vi "ME135_Project_Final.vi"() -> ()   [LabVIEW 2021]
doc: "This example performs writes and reads on a serial port, as directed by the user. You can press the Write and Read buttons, and change the Read Count, while the example is running.\n\nThe parameters set for the serial port must match the parameters of the connected instrument or device. In this example, the Read Count parameter specifies the number of bytes that the serial port reads. If there were more bytes at the port than the specified number, those bytes would not be read. If there were less bytes at the port than the specified number, you would receive a timeout error.\n\nThis example expands upon the flow control options for XON and XOFF, allowing the user to choose those control characters. Also, the user can enable or disable a termination character. Some devices require a termination character in order to identify the end of command strings. Some devices send a termination character to signify the end of data to be read. This example shows how you can end the Read operation once a termination character is detected in the buffer and/or append a termination character at the end of the Write data."
uses:
  Serial - Settings.ctl
  Serial - XON-XOFF Characters.ctl
  Serial - ASCII Characters-1.ctl
  ESP32-PSOC-State Machine.ctl
  <vilib>/Instr/_visa.llb/VISA Flush IO Buffer Mask.ctl
  <vilib>/Instr/_visa.llb/VISA Configure Serial Port (Instr).vi
panel:
  in  "Toggle Motors":bool
  out "Backward":bool
  out "Right":bool
  out "Left":bool
  out "Forward":bool
  out "Obstacle Detected":bool
  out "error":bool=TRUE
  out "Connected":bool
  out "Serial Settings:Number of Bytes at Serial Port":u32
  out "Response 2":string="Exiting LabVIEW"
  in  "Turn On":bool
  in  "Enum":T1
  in  "Termination Character":u8=10 format="%.0x"
  in  "End Write on Termination Character?":bool=TRUE
  in  "Exit Labview":bool
  out "Read Count":u32=1000
  out "Response":string
  in  "XON/XOFF Characters":T2={"XON"=enum."DC1", "XOFF"=enum."DC3"}
  in  "Serial Settings":T4={"baud rate"=115200, "data bits"=8, "parity"=enum."None", "stop bits"=10, "flow control"=0} {"flow control" items=["None"=0, "XON/XOFF"=1, "RTS/CTS"=2, "DTR/DSR"=4]; "stop bits" items=["1.0"=10, "1.5"=15, "2.0"=20]; "data bits" min=5 max=8 step=1; "baud rate" items=["75"=75, "110"=110, "134"=134, "150"=150, "300"=300, "600"=600, "1200"=1200, "1800"=1800, "2400"=2400, "4800"=4800, "7200"=7200, "9600"=9600, "14400"=14400, "19200"=19200, "28800"=28800, "38400"=38400, "56000"=56000, "57600"=57600, "115200"=115200, "128000"=128000, "230400"=230400]}
  in  "End Read on Termination Character?":bool=TRUE
  in  "VISA resource name":refnum<visa-resource-name>="COM8"
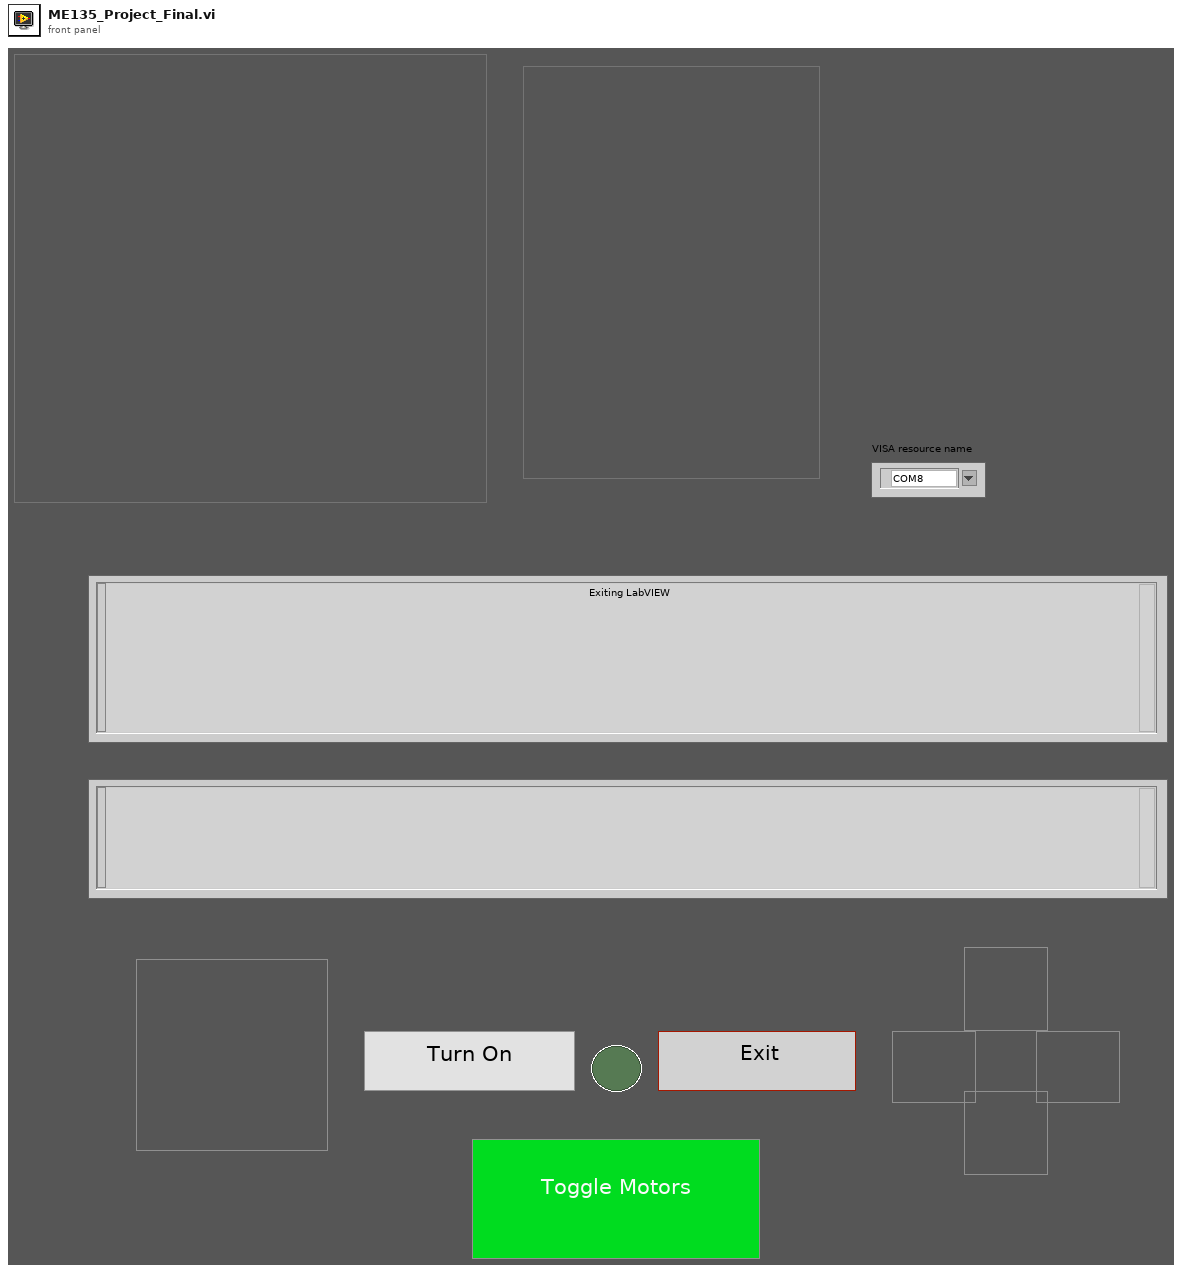
[diagram p1: front panel]
types:
  T1 = typedef "ESP32-PSOC-State Machine.ctl" = enum8{"Init", "Connect", "idle", "send", "wait", "receive", "que", "error", "exit"}
  T2 = typedef "Serial - XON-XOFF Characters.ctl" = cluster{"XON":T3, "XOFF":T3}
  T3 = typedef "Serial - ASCII Characters-1.ctl" = enum16{"NUL", "SOH", "STX", "ETX", "EOT", "ENQ", "ACK", "BEL", "BS", "HT", "LF", "VT", "FF", "CR", "SO", "SI", "DLE", "DC1", "DC2", "DC3", "DC4", "NAK", "SYN", "ETB", "CAN", "EM", "SUB", "ESC", "FS", "GS", "RS", "US", "SP", "!", "\"", "#", "$", "%", "&", "'", "(", ")", "*", "+", ",", "- (-)", ".", "/", "0", "1", "2", "3", "4", "5", "6", "7", "8", "9", ":", ";", "<", "=", ">", "?", "@", "A", "B", "C", "D", "E", "F", "G", "H", "I", "J", "K", "L", "M", "N", "O", "P", "Q", "R", "S", "T", "U", "V", "W", "X", "Y", "Z", "[", "\\", "]", "^", "_", "`", "a", "b", "c", "d", "e", "f", "g", "h", "i", "j", "k", "l", "m", "n", "o", "p", "q", "r", "s", "t", "u", "v", "w", "x", "y", "z", "{", "|", "}", "~"}
  T4 = typedef "Serial - Settings.ctl" = cluster{"baud rate":u32, "data bits":u16, "parity":enum16{"None", "Odd", "Even", "Mark", "Space"}, "stop bits":u16, "flow control":u16}
  T5 = typedef "VISA Flush IO Buffer Mask.ctl" = u16
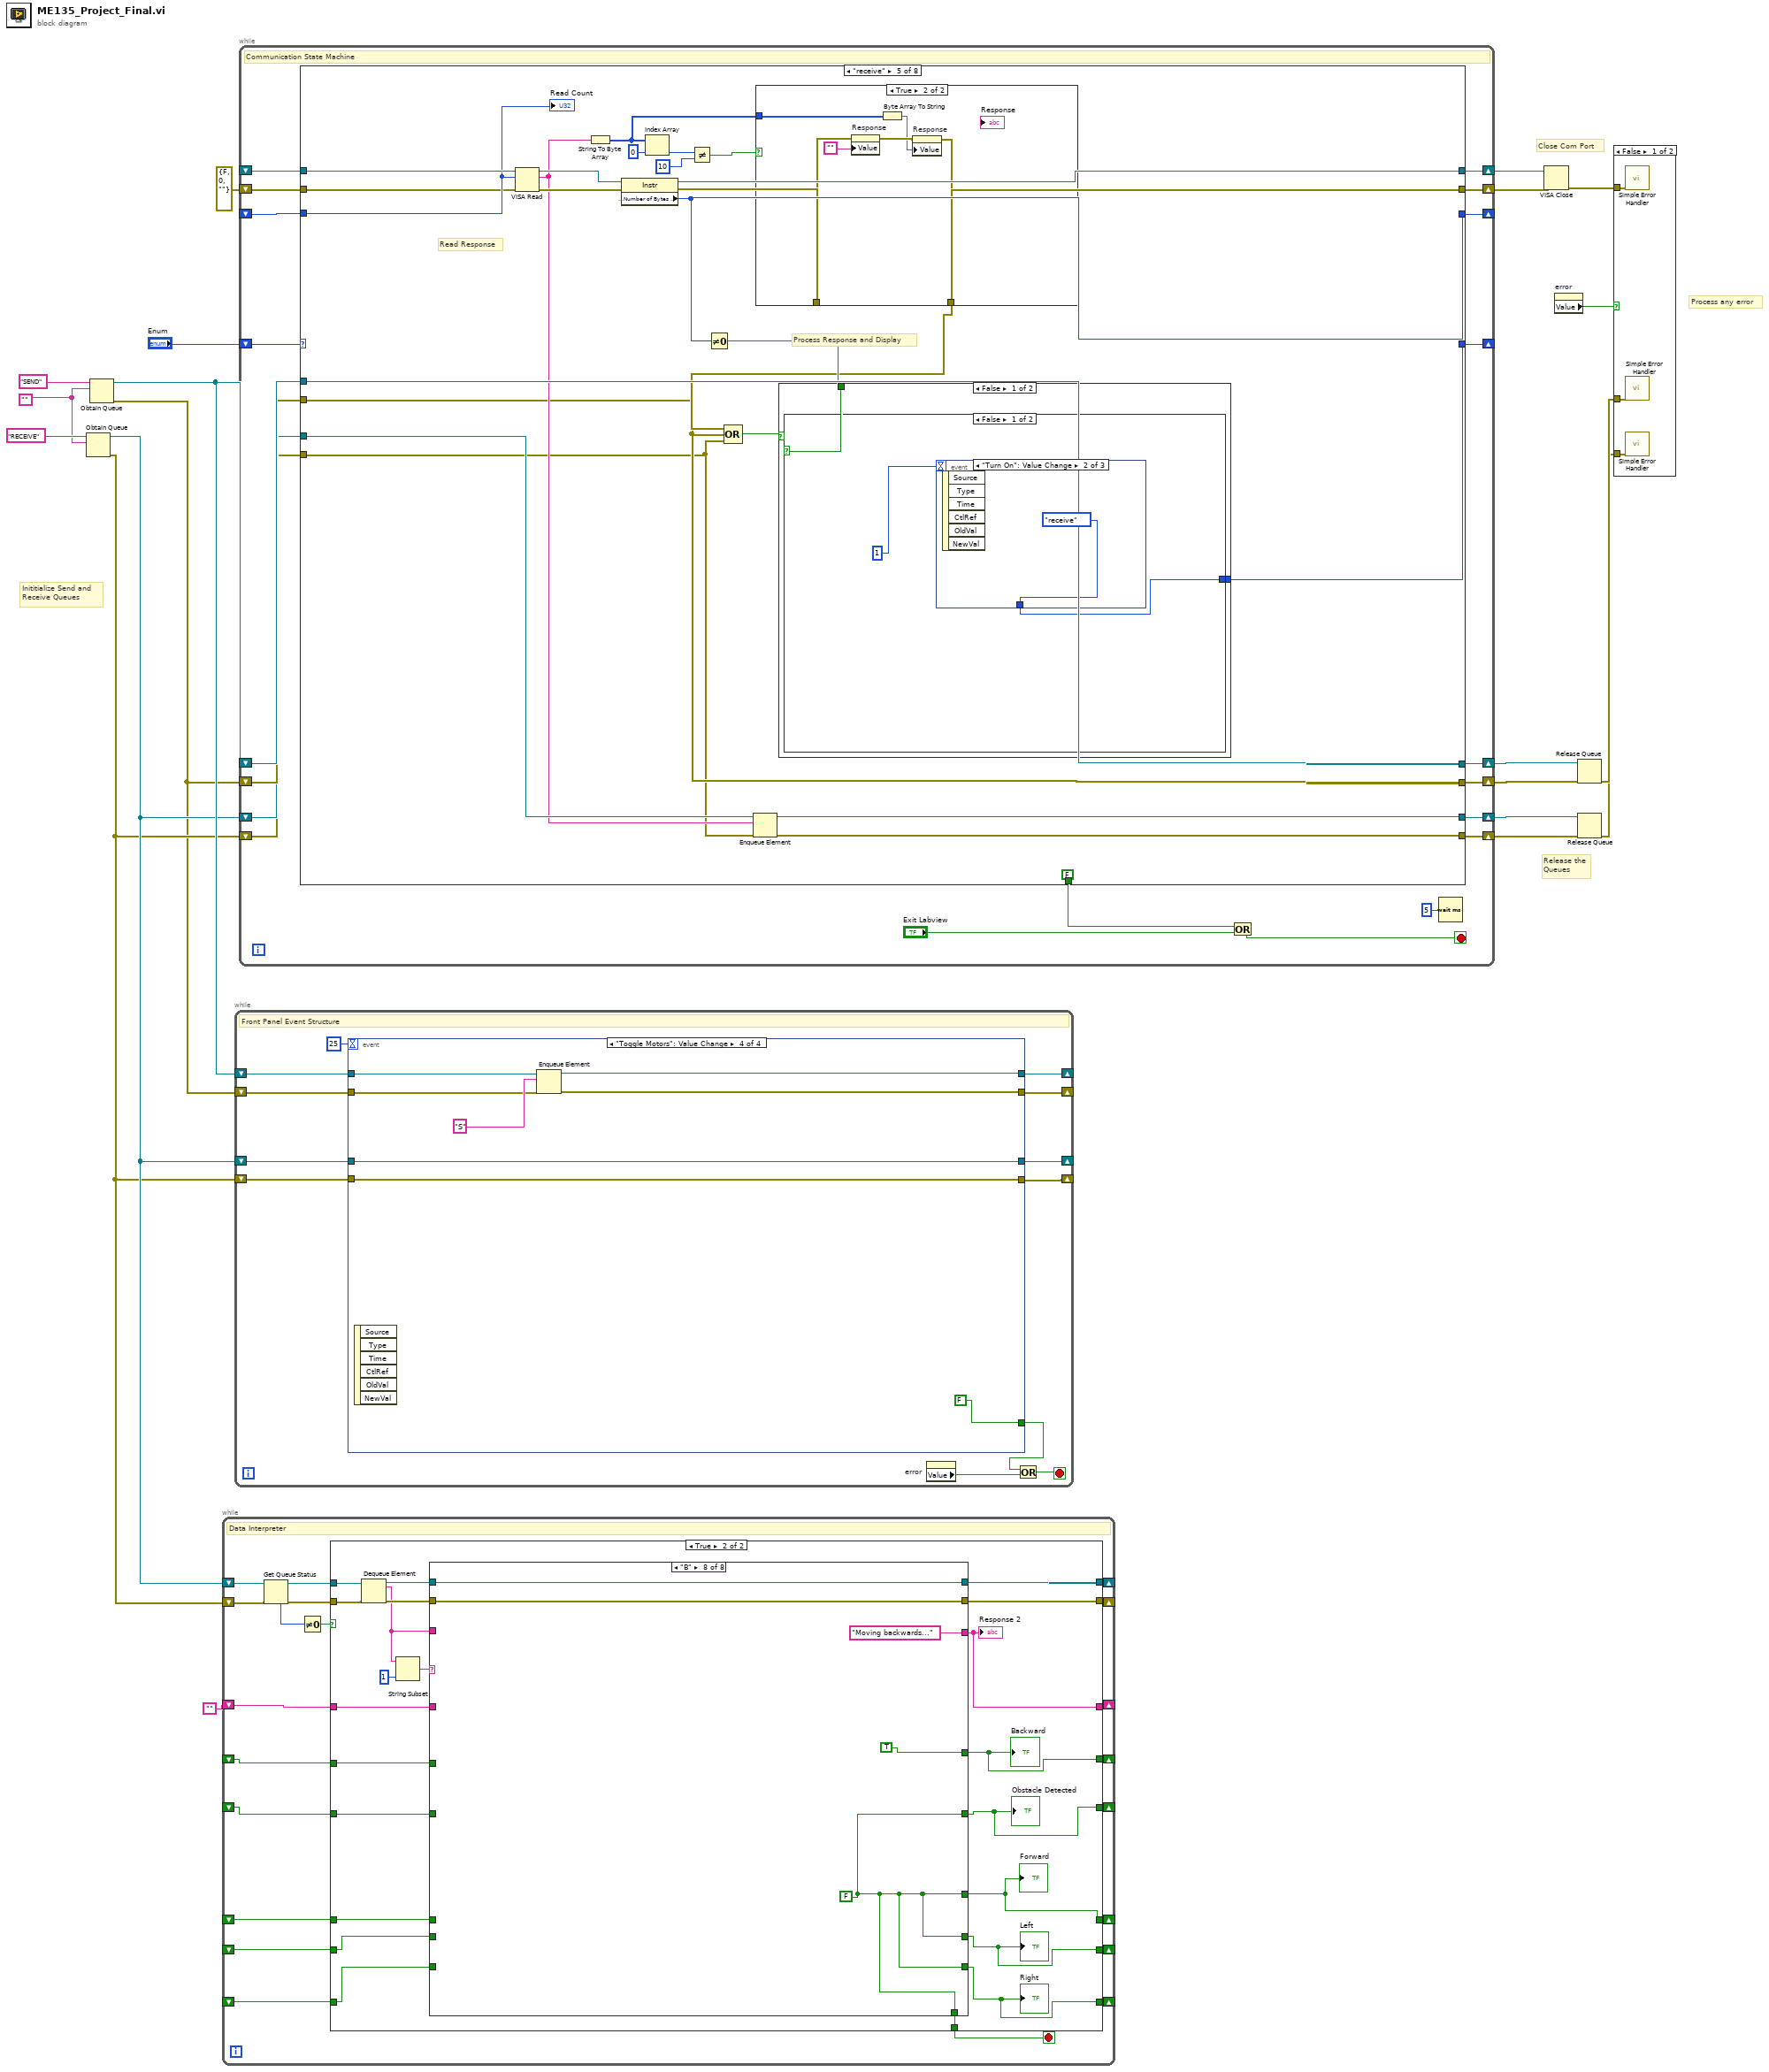
[diagram p0: block diagram]
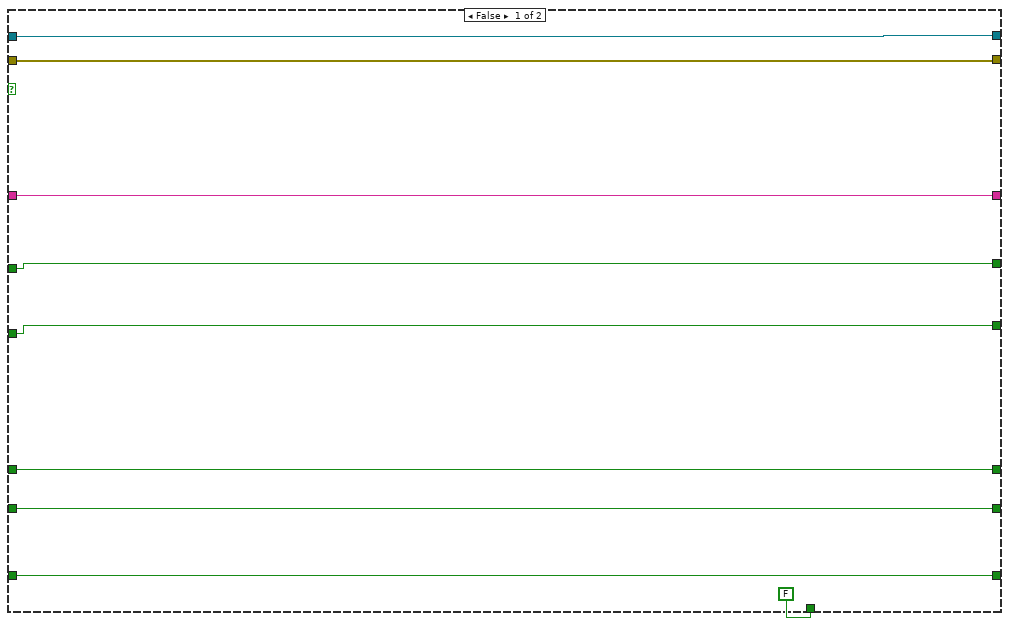
[diagram p3: hidden frame]
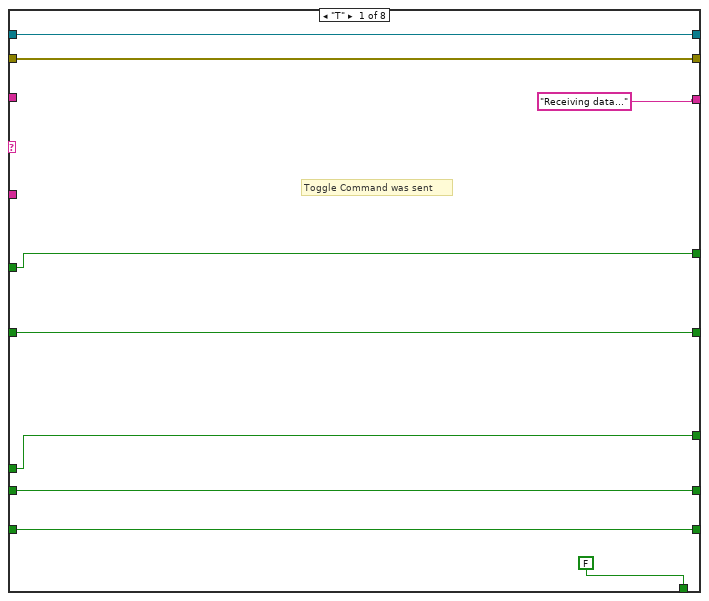
[diagram p4: hidden frame]
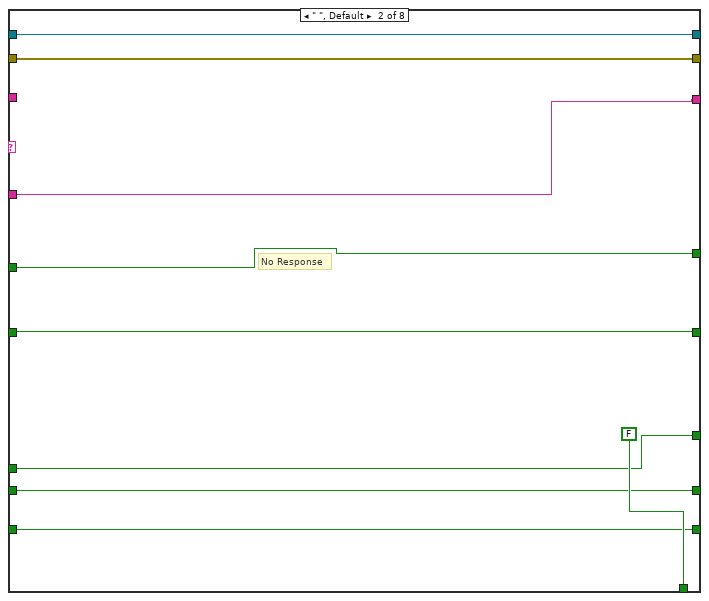
[diagram p5: hidden frame]
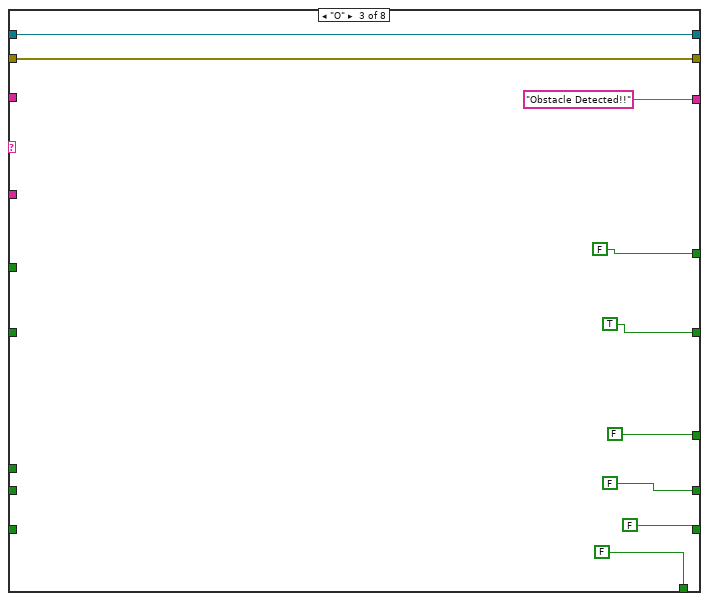
[diagram p6: hidden frame]
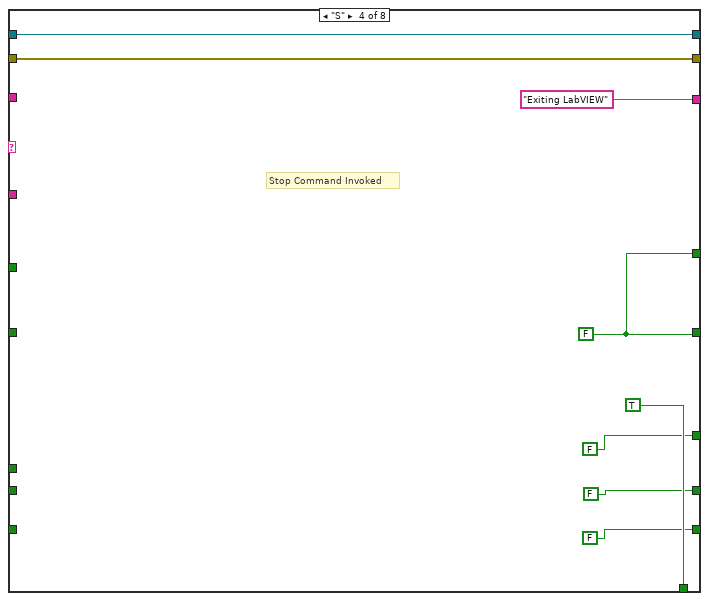
[diagram p7: hidden frame]
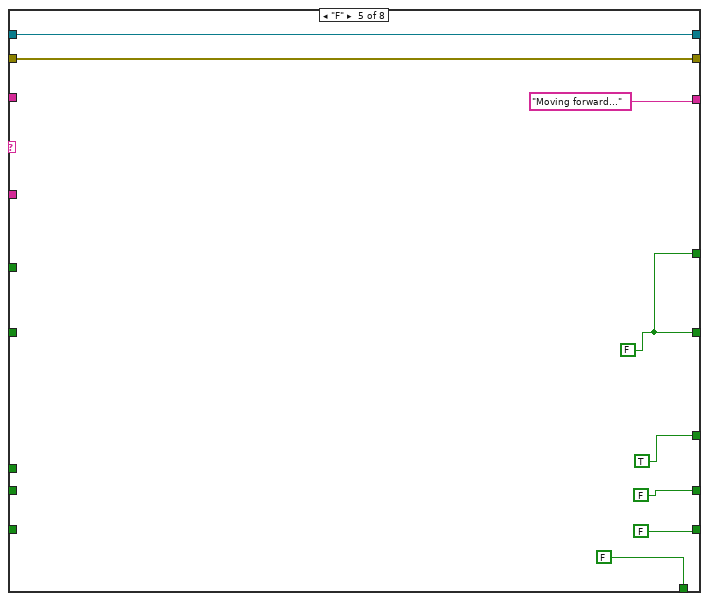
[diagram p8: hidden frame]
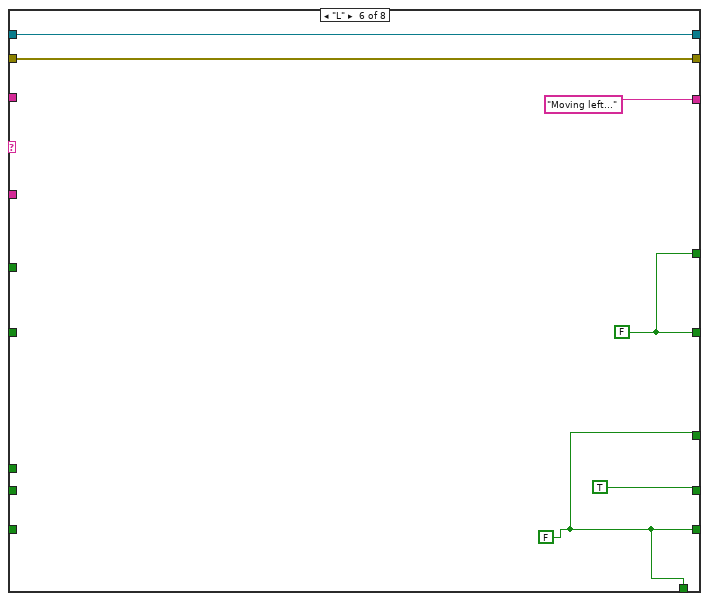
[diagram p9: hidden frame]
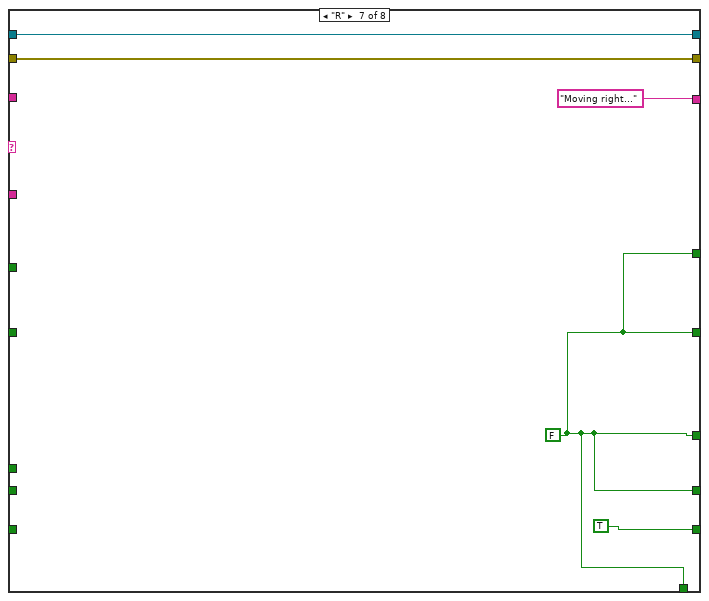
[diagram p10: hidden frame]
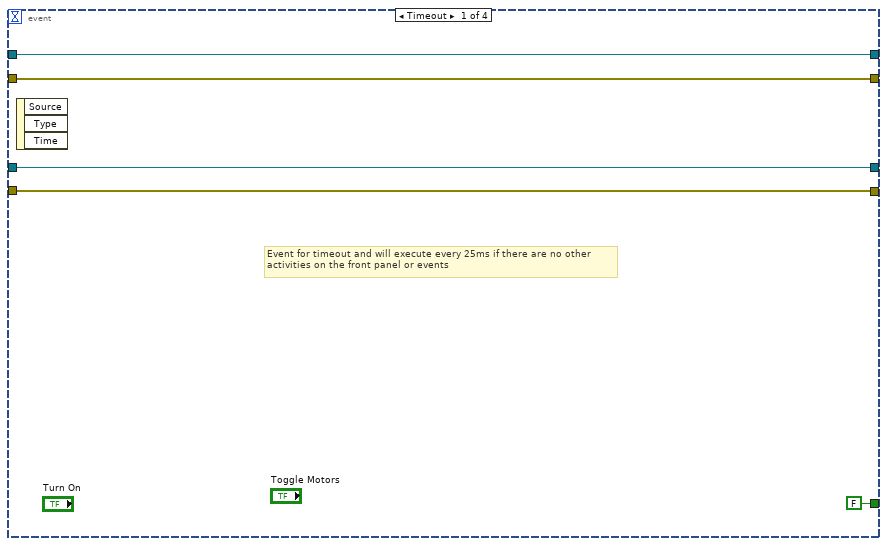
[diagram p11: hidden frame]
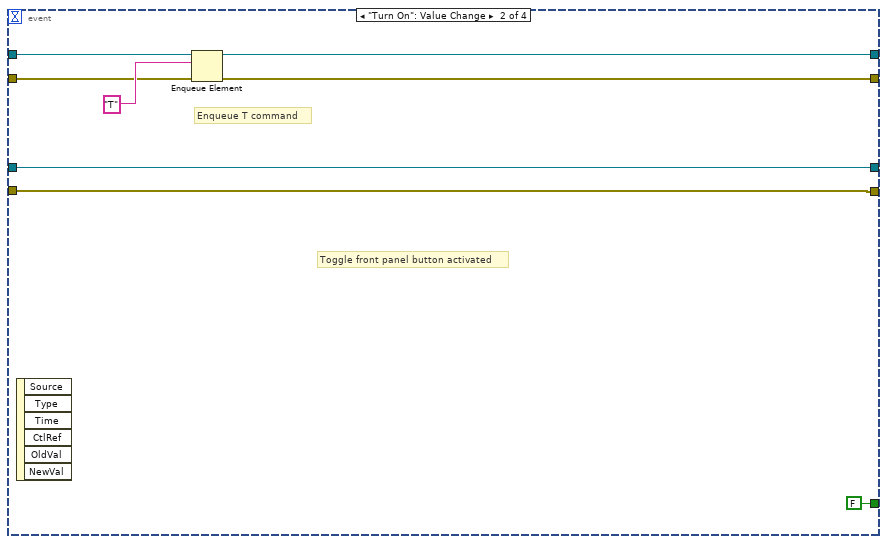
[diagram p12: hidden frame]
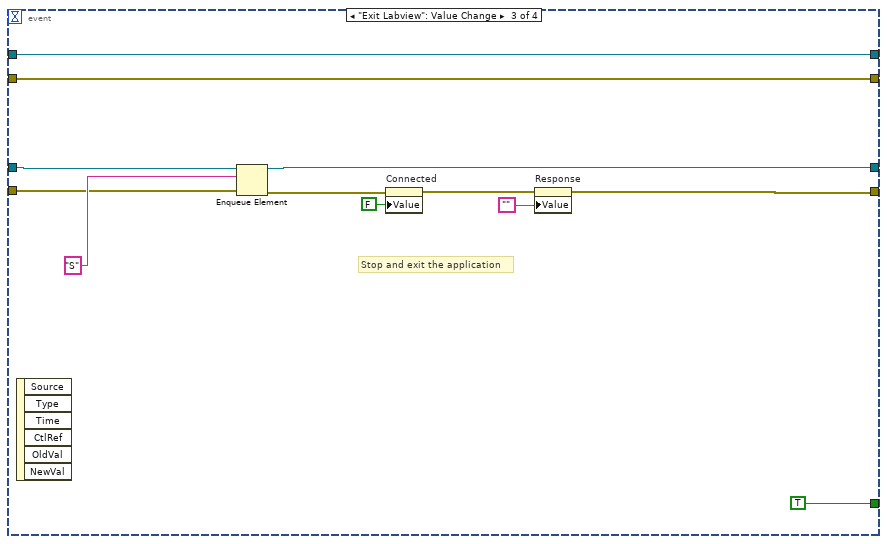
[diagram p13: hidden frame]
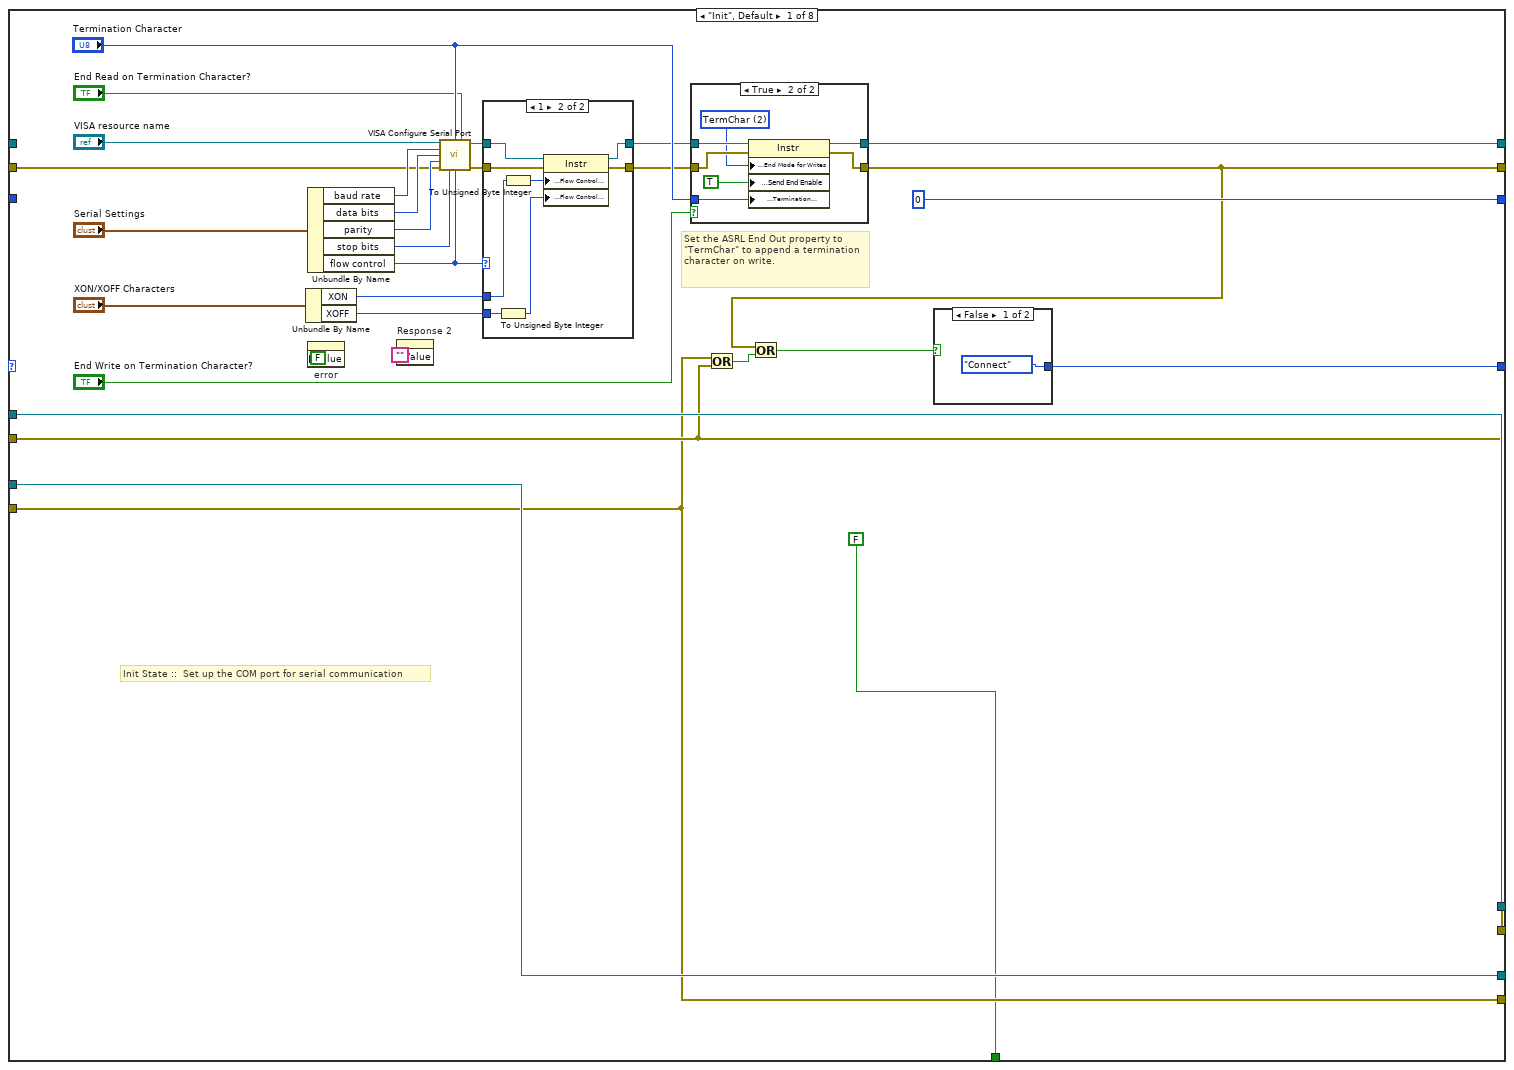
[diagram p14: hidden frame]
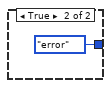
[diagram p15: hidden frame]
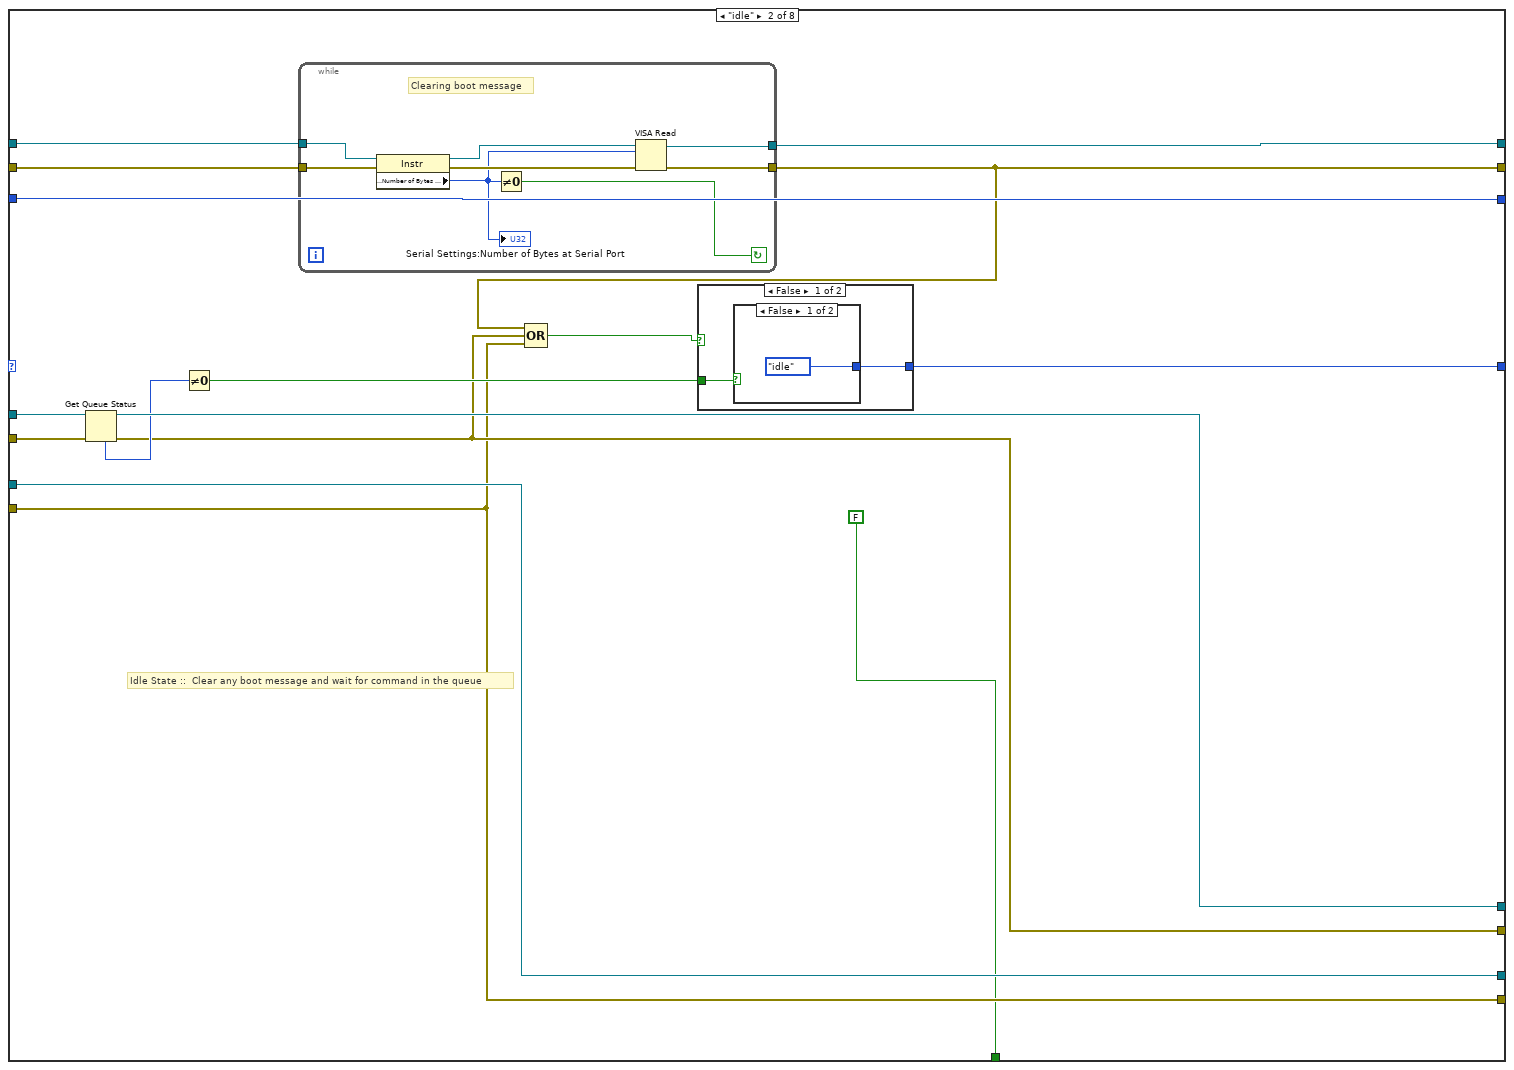
[diagram p18: hidden frame]
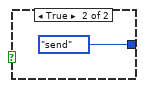
[diagram p19: hidden frame]
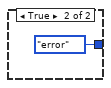
[diagram p20: hidden frame]
diagram:
  w10 = ""
  # "Process any error"
  # "Release the\nQueues"
  # "Close Com Port"
  # "Inititialize Send and\nReceive Queues"
  n1 = Obtain Queue(name (unnamed)="RECEIVE", element data type=w10) -> (queue out=w9:refnum<queue>, error out=w8:errorcluster)  [unwired: 3 in, 1 out]
  n2 = Obtain Queue(name (unnamed)="SEND", element data type=w10) -> (queue out=w12:refnum<queue>, error out=w2:errorcluster)  [unwired: 3 in, 1 out]
  n3 = while {
    shift-right: [w35] -> _
    shift-left: w9 -> [w41]
    shift-right: [w34] -> _
    shift-left: w8 -> [w40]
    shift-right: [w32] -> _
    shift-left: "" -> [w31]
    shift-right: [w29] -> _
    shift-left: _ -> [w30]
    shift-right: [w28] -> _
    shift-left: _ -> [w27]
    shift-right: [w26] -> _
    shift-left: _ -> [w24]
    shift-right: [w25] -> _
    shift-left: _ -> [w23]
    shift-right: [w22] -> _
    shift-left: _ -> [w21]
    stop <- w33 stop-if-true
    # "Data Interpreter"
    n4 = Get Queue Status(queue=w41, error in (no error)=w40) -> (queue out=w37:refnum<queue>, error out=w36:errorcluster, # elements in queue=w39:i32)  [unwired: 1 in, 5 out]
    n5 = Not Equal To 0?(x=w39) -> (x != 0?=w38:bool)
    n6 = case shown="True" w38 {
      tunnel: w37 -> [w50 w72]
      tunnel: w36 -> [w49 w71]
      tunnel: [w50 w66] -> w35
      tunnel: [w49 w65] -> w34
      tunnel: [FALSE w64] -> w33
      tunnel: [w47 w62] -> w32
      tunnel: w31 -> [w47 w61]
      tunnel: w30 -> [w46 w60]
      tunnel: [w46 w59] -> w29
      tunnel: [w45 w58] -> w28
      tunnel: w27 -> [w45 w57]
      tunnel: [w44 w56] -> w26
      tunnel: [w43 w55] -> w25
      tunnel: w24 -> [w44 w54]
      tunnel: w23 -> [w43 w53]
      tunnel: [w42 w52] -> w22
      tunnel: w21 -> [w42 w51]
      frame False {
      }
      frame True {
        n7 = Dequeue Element(queue=w72, error in (no error)=w71) -> (queue out=w70:refnum<queue>, element=w63:string, error out=w69:errorcluster)  [unwired: 1 in, 1 out]
        n8 = String Subset(string=w63, length (rest)=1 ("length (rest)")) -> (substring=w67:string)  [unwired: 1 in]
        n9 = case shown="\"B\"" w67 {
          tunnel: w70 -> [w81 w90 w98 w107 w115 w121 w126 w131]
          tunnel: w69 -> [w80 w89 w97 w106 w114 w120 w125 w130]
          tunnel: [w81 w90 w98 w107 w115 w121 w126 w131] -> w66
          tunnel: [w80 w89 w97 w106 w114 w120 w125 w130] -> w65
          tunnel: w63 -> [_ _ _ _ _ _ _ _]
          tunnel: [FALSE FALSE FALSE TRUE FALSE w118 w122 w128] -> w64
          tunnel: ["Receiving data..." w87 "Obstacle Detected!!" "Exiting LabVIEW" "Moving forward..." "Moving left..." "Moving right..." "Moving backwards..."] -> w62
          tunnel: w61 -> [_ w87 _ _ _ _ _ _]
          tunnel: [w77 w83 TRUE w100 w108 w116 w122 w128] -> w59
          tunnel: w60 -> [w77 w83 _ _ _ _ _ _]
          tunnel: [w76 w86 FALSE FALSE TRUE w118 w122 w128] -> w58
          tunnel: w57 -> [w76 w86 _ _ _ _ _ _]
          tunnel: [w75 w85 FALSE FALSE FALSE TRUE w122 w128] -> w56
          tunnel: [w74 w84 FALSE FALSE FALSE w118 TRUE w128] -> w55
          tunnel: w54 -> [w75 w85 _ _ _ _ _ _]
          tunnel: w53 -> [w74 w84 _ _ _ _ _ _]
          tunnel: [w73 w82 FALSE w100 w108 w116 w122 TRUE] -> w52
          tunnel: w51 -> [w73 w82 _ _ _ _ _ _]
          frame "T" {
            # "Toggle Command was sent"
          }
          frame " ", Default {
            # "No Response"
          }
          frame "O" {
          }
          frame "S" {
            w100 = FALSE
            # "Stop Command Invoked"
          }
          frame "F" {
            w108 = FALSE
          }
          frame "L" {
            w118 = FALSE
            w116 = FALSE
          }
          frame "R" {
            w122 = FALSE
          }
          frame "B" {
            w128 = FALSE
          }
        }
        "Response 2" <- w62
        "Obstacle Detected" <- w59
        "Forward" <- w58
        "Left" <- w56
        "Right" <- w55
        "Backward" <- w52
      }
    }
  }
  n10 = while {
    shift-right: [w140] -> _
    shift-left: w12 -> [w141]
    shift-right: [w139] -> _
    shift-left: w2 -> [w142]
    shift-right: [w135] -> _
    shift-left: w9 -> [w138]
    shift-right: [w136] -> _
    shift-left: w8 -> [w137]
    stop <- w132 stop-if-true
    # "Front Panel Event Structure"
    n11 = event shown="[3] \"Toggle Motors\": Value Change" {
      selector: _ -> [_ _ _ _]
      dyn-events: _ -> [_ _ _ _]
      timeout: 25 -> [_ _ _ _]
      tunnel: w142 -> [w146 w154 w158 w171]
      tunnel: w141 -> [w147 w156 w157 w174]
      tunnel: [w147 w153 w157 w173] -> w140
      tunnel: [w146 w152 w158 w170] -> w139
      tunnel: [FALSE FALSE TRUE FALSE] -> w134
      tunnel: w138 -> [w145 w150 w162 w176]
      tunnel: w137 -> [w144 w149 w160 w175]
      tunnel: [w144 w149 w165 w175] -> w136
      tunnel: [w145 w150 w161 w176] -> w135
      event Timeout {
        # "Event for timeout and will execute every 25ms if there are no other\nactivities on the front panel or events"
        n12 = event-data() -> ()  [unwired: 1 in, 3 out]
      }
      event "Turn On": Value Change {
        # "Enqueue T command"
        # "Toggle front panel button activated"
        n13 = event-data() -> ()  [unwired: 1 in, 6 out]
        n14 = Enqueue Element(queue=w156, element="T", error in (no error)=w154) -> (queue out=w153:refnum<queue>, error out=w152:errorcluster)  [unwired: 1 in, 1 out]
      }
      event "Exit Labview": Value Change {
        # "Stop and exit the application"
        n15 = event-data() -> ()  [unwired: 1 in, 6 out]
        n16 = Enqueue Element(queue=w162, element="S", error in (no error)=w160) -> (queue out=w161:refnum<queue>, error out=w159:errorcluster)  [unwired: 1 in, 1 out]
        n17 = property on="Connected" class="Bool (strict)"(error in=w159, "Value"=FALSE ("Connected")) -> (error out=w166:errorcluster)  [unwired: 1 in, 1 out]
        n18 = property on="Response" class="Str"(error in=w166, "Value"="") -> (error out=w165:errorcluster)  [unwired: 1 in, 1 out]
      }
      event "Toggle Motors": Value Change {
        n19 = event-data() -> ()  [unwired: 1 in, 6 out]
        n20 = Enqueue Element(queue=w174, element="S", error in (no error)=w171) -> (queue out=w173:refnum<queue>, error out=w170:errorcluster)  [unwired: 1 in, 1 out]
      }
    }
    n21 = property on="error" class="Bool (strict)"() -> ("Value"=w133:bool)  [unwired: 2 in, 2 out]
    n22 = Or(x=w134, y=w133) -> (x .or. y?=w132:bool)
  }
  n23 = while {
    shift-right: [w188] -> w20
    shift-left: w12 -> [w196]
    shift-right: [w187] -> w18
    shift-left: w2 -> [w195]
    shift-right: [w186] -> w19
    shift-left: w9 -> [w194]
    shift-right: [w185] -> w15
    shift-left: w8 -> [w193]
    shift-right: [w180] -> _
    shift-left: "Enum" -> [w179]
    shift-right: [w192] -> w14
    shift-left: _ -> [w189]
    shift-right: [w191] -> w13
    shift-left: errorcluster {"status"=FALSE, "code"=0, "source"=""} ("error out") -> [w190]
    shift-right: [w184] -> _
    shift-left: _ -> [w183]
    stop <- w178 stop-if-true
    # "Communication State Machine"
    n24 = case shown="\"receive\"" w179 {
      selector: w179 -> [_ _ _ _ _ _ w381 _]
      tunnel: [w226 w262 w293 w306 w339 w365 w380 w390] -> w188
      tunnel: [w200 w252 w281 w300 w319 w362 w379 w389] -> w187
      tunnel: [w206 w260 w283 w310 w340 ESP32-PSOC-State_Machine."exit" ("Enum") w381 w386] -> w180
      tunnel: w196 -> [w226 w264 w295 w306 w339 w365 w380 w390]
      tunnel: w195 -> [w200 w263 w294 w300 w319 w362 w379 w389]
      tunnel: w194 -> [w227 w258 w290 w303 w334 w364 w378 w388]
      tunnel: w193 -> [w199 w251 w280 w299 w318 w361 w369 w387]
      tunnel: [w208 w255 w291 w308 w329 w367 w384 w393] -> w192
      tunnel: [w202 w253 w282 w301 w320 w363 w383 w394] -> w191
      tunnel: w190 -> [w204 w254 w286 w307 w322 w363 w383 w395]
      tunnel: w189 -> [_ w256 w288 w309 w337 w367 w384 w396]
      tunnel: [w227 w258 w290 w303 w332 w364 w376 w388] -> w186
      tunnel: [w199 w251 w280 w299 w333 w361 w372 w387] -> w185
      tunnel: [u32 0 ("Bytes at Port") w257 w289 w305 w335 w366 w382 w391] -> w184
      tunnel: w183 -> [_ w257 w289 _ w331 w366 w382 w392]
      tunnel: [FALSE FALSE FALSE FALSE FALSE FALSE TRUE FALSE] -> w177
      frame "Init", Default {
        # "Init State ::  Set up the COM port for serial communication"
        # "Set the ASRL End Out property to \"TermChar\" to append a termination character on write."
        n25 = Unbundle By Name("XON/XOFF Characters") -> ("XON"=w220:T3, "XOFF"=w221:T3)
        n26 = Unbundle By Name("Serial Settings") -> ("baud rate"=w216:u32, "data bits"=w215:u16, "parity"=w214:enum16{"None", "Odd", "Even", "Mark", "Space"}, "stop bits"=w213:u16, "flow control"=w219:u16)
        n27 = property on="error" class="Bool (strict)"("Value"=FALSE ("error")) -> ()  [unwired: 2 in, 2 out]
        n28 = property on="Response 2" class="Str"("Value"="") -> ()  [unwired: 2 in, 2 out]
        n29 = call-poly "VISA Configure Serial Port"("VISA resource name"="VISA resource name", "termination char\n(0xA = '\\n' = LF)"="Termination Character", "Enable Termination\nChar (T)"="End Read on Termination Character?", "baud rate (9600)"=w216, "data bits (8)"=w215, "parity (0:none)"=w214, "error in (no error)"=w204, "stop bits (10: 1 bit)"=w213, "flow control (0:none)"=w219) -> ("VISA resource name out"=w212:refnum<visa-resource-name>, "error out"=w211:errorcluster)  [unwired: 1 in, 4 out]
        n30 = case shown="1" w219 {
          tunnel: [w239 w248] -> w222
          tunnel: [w240 w247] -> w223
          tunnel: w211 -> [w239 w246]
          tunnel: w212 -> [w240 w245]
          tunnel: w220 -> [_ w244]
          tunnel: w221 -> [_ w243]
          frame Default {
          }
          frame 1 {
            n31 = To Unsigned Byte Integer(number=w243) -> (unsigned 8bit integer=w242:u8)
            n32 = To Unsigned Byte Integer(number=w244) -> (unsigned 8bit integer=w241:u8)
            n33 = property class="Instr"(reference=w245, error in=w246, "Serial Settings:Flow Control XON Character"=w241, "Serial Settings:Flow Control XOFF Character"=w242) -> (reference out=w247:refnum<visa-resource-name>, error out=w248:errorcluster)
          }
        }
        n34 = case shown="True" "End Write on Termination Character?" {
          tunnel: w223 -> [w230 w238]
          tunnel: w222 -> [w231 w237]
          tunnel: [w230 w236] -> w208
          tunnel: [w231 w235] -> w202
          tunnel: "Termination Character" -> [_ w233]
          frame False {
          }
          frame True {
            w234 = u16 2 items=["None", "LastBit", "TermChar", "Break"] ("Serial Settings:Serial End Mode for Writes")
            n35 = property class="Instr"(reference=w238, error in=w237, "Serial Settings:End Mode for Writes"=w234, "Message Based Settings:Send End Enable"=TRUE, "Message Based Settings:Termination Character"=w233) -> (reference out=w236:refnum<visa-resource-name>, error out=w235:errorcluster)
          }
        }
        n36 = Or(x=w199, y=w200) -> (x .or. y?=w201:bool)
        n37 = Or(x=w202, y=w201) -> (x .or. y?=w203:bool)
        n38 = case shown="False" w203 {
          tunnel: [ESP32-PSOC-State_Machine."Connect" ("Enum") ESP32-PSOC-State_Machine."error" ("Enum")] -> w206
          frame False {
          }
          frame True {
          }
        }
      }
      frame "idle" {
        # "Idle State ::  Clear any boot message and wait for command in the queue"
        n39 = Get Queue Status(queue=w264, error in (no error)=w263) -> (queue out=w262:refnum<queue>, error out=w252:errorcluster, # elements in queue=w261:i32)  [unwired: 1 in, 5 out]
        n40 = Not Equal To 0?(x=w261) -> (x != 0?=w259:bool)
        n41 = while {
          tunnel: w256 -> [w277]
          tunnel: [w273] -> w255
          tunnel: w254 -> [w276]
          tunnel: [w271] -> w253
          stop <- w275 continue-if-true
          # "Clearing boot message"
          n42 = property class="Instr"(reference=w277, error in=w276) -> (reference out=w274:refnum<visa-resource-name>, error out=w272:errorcluster, "Serial Settings:Number of Bytes at Serial Port"=w270:u32)
          "Serial Settings:Number of Bytes at Serial Port" <- w270
          n43 = Not Equal To 0?(x=w270) -> (x != 0?=w275:bool)
          n44 = VISA Read(VISA resource name=w274, byte count=w270, error in (no error)=w272) -> (VISA resource name out=w273:refnum<visa-resource-name>, error out=w271:errorcluster)  [unwired: 2 out]
        }
        n45 = Compound Arithmetic op=OR(w253, w252, w251) -> (w250:bool)
        n46 = case shown="False" w250 {
          tunnel: [w266 ESP32-PSOC-State_Machine."error" ("Enum")] -> w260
          tunnel: w259 -> [w265 _]
          frame False {
            n47 = case shown="False" w265 {
              tunnel: [ESP32-PSOC-State_Machine."idle" ("Enum") ESP32-PSOC-State_Machine."send" ("Enum")] -> w266
              frame False {
              }
              frame True {
              }
            }
          }
          frame True {
          }
        }
      }
      frame "send" {
        w284 = T5 64 items=["Flush Receive Buffer"=16, "Write Transmit Buffer to Device"=32, "Flush Receive Buffer (No I/O)"=64, "Flush Transmit Buffer"=128] ("Mask")
        # "Send the command"
        # "Clear the receive buffer for new message"
        n48 = Dequeue Element(queue=w295, error in (no error)=w294) -> (queue out=w293:refnum<queue>, element=w292:string, error out=w281:errorcluster)  [unwired: 1 in, 1 out]
        n49 = VISA Flush I/O Buffer(VISA resource name=w288, mask (16)=w284, error in (no error)=w286) -> (VISA resource name out=w287:refnum<visa-resource-name>, error out=w285:errorcluster)
        n50 = VISA Write(VISA resource name=w287, write buffer=w292, error in (no error)=w285) -> (VISA resource name out=w291:refnum<visa-resource-name>, error out=w282:errorcluster)  [unwired: 1 out]
        n51 = Compound Arithmetic op=OR(w282, w281, w280) -> (w279:bool)
        n52 = case shown="False" w279 {
          tunnel: [ESP32-PSOC-State_Machine."wait" ("Enum") ESP32-PSOC-State_Machine."error" ("Enum")] -> w283
          frame False {
          }
          frame True {
          }
        }
      }
      frame "wait" {
        # "Wait for Response"
        n53 = property class="Instr"(reference=w309, error in=w307) -> (reference out=w308:refnum<visa-resource-name>, error out=w301:errorcluster, "Serial Settings:Number of Bytes at Serial Port"=w305:u32)
        n54 = Not Equal To 0?(x=w305) -> (x != 0?=w304:bool)
        n55 = Compound Arithmetic op=OR(w301, w300, w299) -> (w302:bool)
        n56 = case shown="False" w302 {
          tunnel: [w312 ESP32-PSOC-State_Machine."Connect" ("Enum")] -> w310
          tunnel: w304 -> [w311 _]
          frame False {
            n57 = case shown="False" w311 {
              tunnel: [ESP32-PSOC-State_Machine."receive" ("Enum") ESP32-PSOC-State_Machine."receive" ("Enum")] -> w312
              frame False {
              }
              frame True {
              }
            }
          }
          frame True {
          }
        }
      }
      frame "receive" {
        # "Process Response and Display"
        # "Read Response"
        n58 = VISA Read(VISA resource name=w337, byte count=w331, error in (no error)=w322) -> (VISA resource name out=w330:refnum<visa-resource-name>, read buffer=w325:string, error out=w336:errorcluster)  [unwired: 1 out]
        n59 = String To Byte Array(string=w325) -> (unsigned byte array=w323:u8[])
        n60 = property class="Instr"(reference=w330, error in=w336) -> (reference out=w329:refnum<visa-resource-name>, error out=w321:errorcluster, "Serial Settings:Number of Bytes at Serial Port"=w335:u32)
        n61 = Index Array(array=w323, index=0) -> (element=w327:u8)
        n62 = Not Equal?(x=w327, y=u8 10) -> (x != y?=w324:bool)
        n63 = Not Equal To 0?(x=w335) -> (x != 0?=w338:bool)
        n64 = Enqueue Element(queue=w334, element=w325, error in (no error)=w318) -> (queue out=w332:refnum<queue>, error out=w333:errorcluster)  [unwired: 1 in, 1 out]
        n65 = case shown="True" w324 {
          tunnel: w323 -> [_ w351]
          tunnel: w321 -> [w350 w353]
          tunnel: [w350 w352] -> w320
          frame False {
          }
          frame True {
            n66 = property on="Response" class="Str"(error in=w353, "Value"="") -> (error out=w355:errorcluster)  [unwired: 1 in, 1 out]
            n67 = Byte Array To String(unsigned byte array=w351) -> (string=w354:string)
            n68 = property on="Response" class="Str"(error in=w355, "Value"=w354) -> (error out=w352:errorcluster)  [unwired: 1 in, 1 out]
          }
        }
        n69 = Compound Arithmetic op=OR(w320, w319, w318) -> (w317:bool)
        n70 = case shown="False" w317 {
          tunnel: [w341 ESP32-PSOC-State_Machine."error" ("Enum")] -> w340
          tunnel: w338 -> [w342 _]
          frame False {
            n71 = case shown="False" w342 {
              tunnel: [w343 ESP32-PSOC-State_Machine."receive" ("Enum")] -> w341
              frame False {
                n72 = event shown="[1] \"Turn On\": Value Change" {
                  selector: _ -> [_ _ _]
                  dyn-events: _ -> [_ _ _]
                  timeout: 1 -> [_ _ _]
                  tunnel: [ESP32-PSOC-State_Machine."receive" ("Enum") ESP32-PSOC-State_Machine."receive" ("Enum") ESP32-PSOC-State_Machine."send" ("Enum")] -> w343
                  event Timeout {
                    n73 = event-data() -> ()  [unwired: 1 in, 3 out]
                  }
                  event "Turn On": Value Change {
                    n74 = event-data() -> ()  [unwired: 1 in, 6 out]
                  }
                  event "Toggle Motors": Value Change {
                    n75 = event-data() -> ()  [unwired: 1 in, 6 out]
                  }
                }
              }
              frame True {
              }
            }
          }
          frame True {
          }
        }
        "Read Count" <- w331
      }
      frame "error" {
        # "Processing Errors"
        n76 = Build Array(w363, w362, w361) -> (w360:errorcluster[])
        n77 = for {
          tunnel: w360 -> [w368] mode=indexing
          n78 = call <vilib>:"General Error Handler.vi"("error in (no error)"=w368) -> ()  [unwired: 10 in, 5 out]
        }
        "error" <- TRUE ("error")
      }
      frame "exit" {
        # "Stop execution due to error"
        n79 = Enqueue Element(queue=w378, element="S", error in (no error)=w369) -> (queue out=w376:refnum<queue>, error out=w374:errorcluster)  [unwired: 1 in, 1 out]
        n80 = property on="Connected" class="Bool (strict)"(error in=w374, "Value"=FALSE ("Connected")) -> (error out=w373:errorcluster)  [unwired: 1 in, 1 out]
        n81 = property on="Response" class="Str"(error in=w373, "Value"="") -> (error out=w372:errorcluster)  [unwired: 1 in, 1 out]
      }
      frame "Connect" {
        n82 = while {
          shift-right: [w409] -> w394
          shift-left: w395 -> [w416]
          shift-right: [w411] -> w393
          shift-left: w396 -> [w417]
          tunnel: w392 -> [w398]
          tunnel: [w398] -> w391
          tunnel: [ESP32-PSOC-State_Machine."idle" ("Enum")] -> w386
          i -> [w403]
          stop <- w399 stop-if-true
          n83 = VISA Write(VISA resource name=w417, write buffer="I", error in (no error)=w416) -> (VISA resource name out=w413:refnum<visa-resource-name>, error out=w414:errorcluster)  [unwired: 1 out]
          n84 = while {
            shift-right: [w423] -> w410
            shift-left: w414 -> [w424]
            shift-right: [w421] -> w412
            shift-left: w413 -> [w422]
            tunnel: [w418] -> w408
            stop <- w420 continue-if-true
            n85 = property class="Instr"(reference=w422, error in=w424) -> (reference out=w421:refnum<visa-resource-name>, error out=w423:errorcluster, "Bytes at Port"=w418:u32)
            n86 = Wait (ms)(milliseconds to wait=u32 5) -> ()  [unwired: 1 out]
            n87 = Equal To 0?(x=w418) -> (x = 0?=w420:bool)
          }
          n88 = VISA Read(VISA resource name=w412, byte count=w408, error in (no error)=w410) -> (VISA resource name out=w411:refnum<visa-resource-name>, read buffer=w407:string, error out=w409:errorcluster)  [unwired: 1 out]
          n89 = Search/Split String(string=w407, search string/char (-)="IPSOC") -> (match + rest of string=w405:string)  [unwired: 1 in, 2 out]
          n90 = String Length(string=w405) -> (length=w404:i32)
          n91 = Not Equal To 0?(x=w404) -> (x != 0?=w401:bool)
          n92 = Greater?(x=w403, y=5) -> (0:w400:bool)
          n93 = And(x=w401, y=w400) -> (x .and. y?=w399:bool)
          "Connected" <- w399
        }
      }
    }
    n94 = Or(x=w177, y="Exit Labview") -> (x .or. y?=w178:bool)
    n95 = Wait (ms)(milliseconds to wait=u32 5) -> ()  [unwired: 1 out]
  }
  n96 = VISA Close(VISA resource name=w14, error in (no error)=w13) -> (error out=w5:errorcluster)
  n97 = property on="error" class="Bool (strict)"() -> ("Value"=w1:bool)  [unwired: 2 in, 2 out]
  n98 = Release Queue(queue=w20, error in (no error)=w18) -> (error out=w4:errorcluster)  [unwired: 1 in, 2 out]
  n99 = Release Queue(queue=w19, error in (no error)=w15) -> (error out=w3:errorcluster)  [unwired: 1 in, 2 out]
  n100 = case shown="False" w1 {
    tunnel: w5 -> [w427 _]
    tunnel: w4 -> [w426 _]
    tunnel: w3 -> [w425 _]
    frame False {
      n101 = call <vilib>:"Simple Error Handler.vi"("error in (no error)"=w427) -> ()  [unwired: 1 in, 8 out]
      n102 = call <vilib>:"Simple Error Handler.vi"("error in (no error)"=w426) -> ()  [unwired: 1 in, 8 out]
      n103 = call <vilib>:"Simple Error Handler.vi"("error in (no error)"=w425) -> ()  [unwired: 1 in, 8 out]
    }
    frame True {
    }
  }
